vi "例13.3-1过零法.vi"() -> ()   [LabVIEW 2017]
panel:
  out "频率":dbl
  in  "信噪比":dbl=1.0 format="%.2p"
  in  "相位":dbl
  in  "采样信息":cluster{"Fs":dbl, "#s":dbl}={"Fs"=1000.0, "#s"=1000.0}
  in  "幅值":dbl=1.0
  in  "频率":dbl=10.5
  in  "噪声选择":enum16{"无", "均匀白噪声", "高斯噪声"}(ring)
  out "波形图":waveform(dbl)(graph)
  # "过零法测量结果"
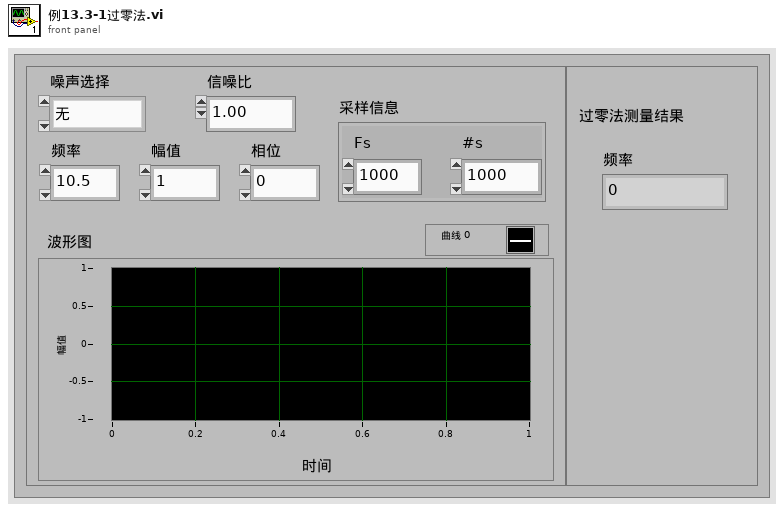
[diagram p1: front panel]
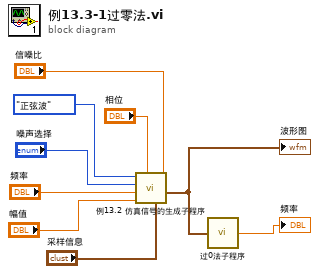
[diagram p0: block diagram]
diagram:
  n1 = call "例13.2 仿真信号的生成子程序.vi"("信噪比"="信噪比", "sampling info"="采样信息", "相位"="相位", "幅值"="幅值", "频率"="频率", "噪声选择"="噪声选择", "波形选择"=enum16{"正弦波", "三角波", "方波", "公式波"}."正弦波") -> ("波形图"=w3:waveform(dbl))  [unwired: 4 in]
  "波形图" <- w3
  n2 = call "过0法子程序.vi"("波形"=w3) -> ("f"=→"频率":dbl)
